vi "Set Colour.vi"(0 "Quick-GUI-Update in":refnum<class "Quick-GUI-Update.lvclass">, 2 "Label":string, 5 "Outer Color":u32(colorbox)=12369084, 9 "Inner Color":u32(colorbox), 11 "Error In":errorcluster) -> (4 "Quick-GUI-Update out":refnum<class "Quick-GUI-Update.lvclass">, 15 "Error Out":errorcluster)   [LabVIEW 2020, in "Easy GUI Operation.lvlib" / "Quick-GUI-Update.lvclass"]
uses:
  Quick-GUI-Update.lvclass
  Quick-GUI-Update.lvclass/Quick-GUI-Update.ctl
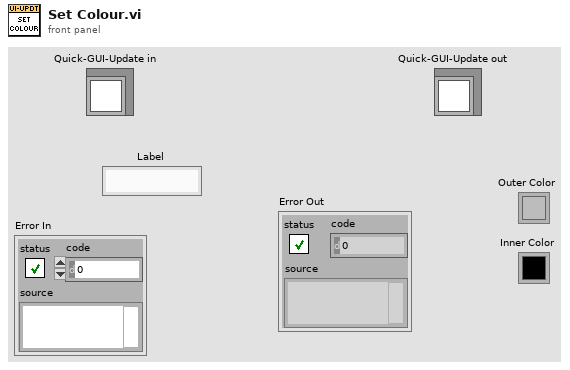
[diagram p1: front panel]
types:
  T1 = map{string, set{cluster{"Ctrl-Ref":refnum<vi>, "Ctrl Index":i32, "Class-Name":string, "Class ID":u32}}}
  T2 = set{cluster{"Ctrl-Ref":refnum<vi>, "Ctrl Index":i32, "Class-Name":string, "Class ID":u32}}
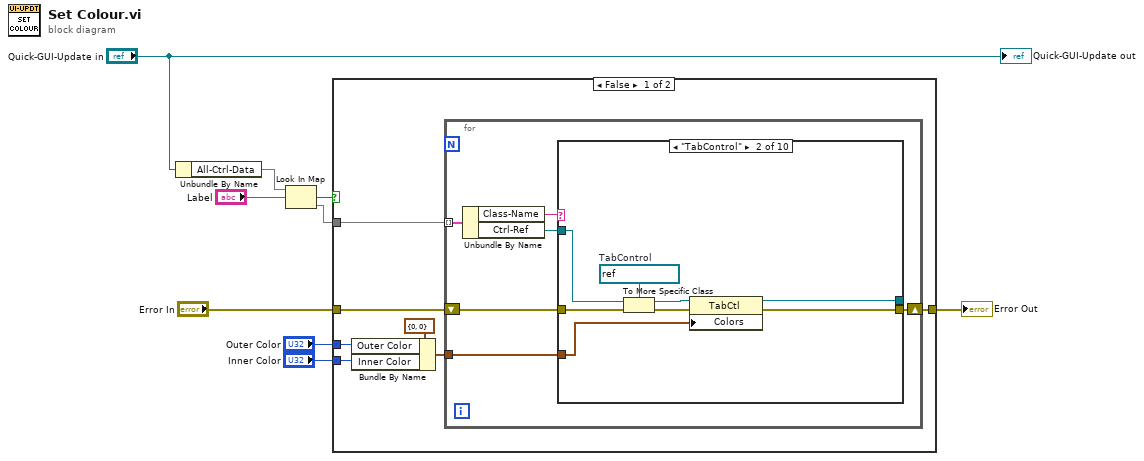
[diagram p0: block diagram]
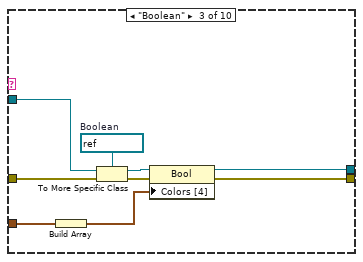
[diagram p3: hidden frame]
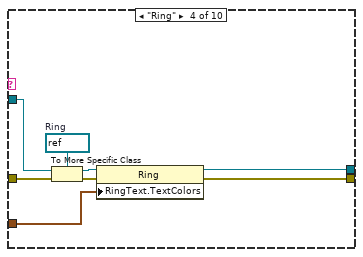
[diagram p4: hidden frame]
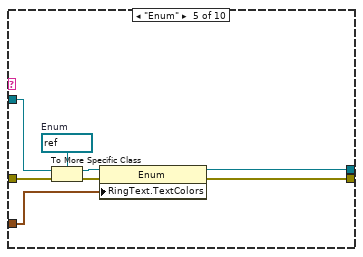
[diagram p5: hidden frame]
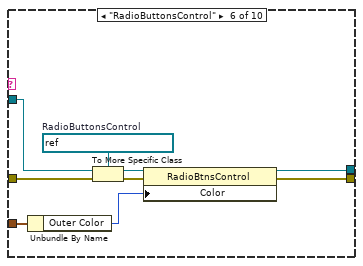
[diagram p6: hidden frame]
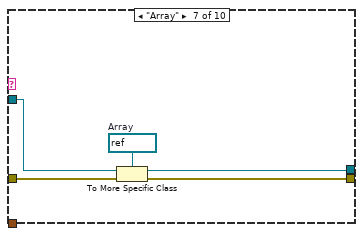
[diagram p7: hidden frame]
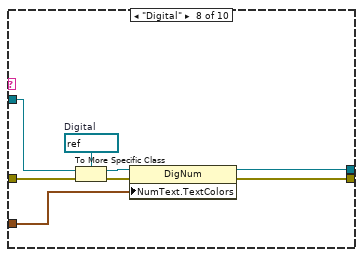
[diagram p8: hidden frame]
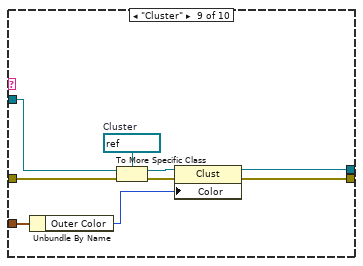
[diagram p9: hidden frame]
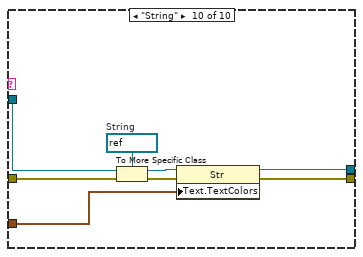
[diagram p10: hidden frame]
diagram:
  n1 = Unbundle By Name("Quick-GUI-Update in") -> ("All-Ctrl-Data"=w4:T1)
  n2 = Look In Map(map=w4, key="Label") -> (key not found?=w1:bool, value=w2:T2)  [unwired: 1 in]
  n3 = case shown="False" w1 {
    tunnel: "Error In" -> [w16 w94]
    tunnel: [w15 w94] -> w8
    tunnel: "Outer Color" -> [w12 _]
    tunnel: "Inner Color" -> [w11 _]
    tunnel: w2 -> [w14 _]
    frame False {
      n4 = Bundle By Name(cluster=cluster{"Outer Color":u32, "Inner Color":u32} {"Outer Color"=0, "Inner Color"=0} ("Color"), "Outer Color"=w12, "Inner Color"=w11) -> (w10:cluster{"Outer Color":u32, "Inner Color":u32})
      n5 = for {
        shift-right: [w21] -> w15
        shift-left: w16 -> [w22]
        tunnel: w14 -> [w20] mode=indexing
        tunnel: w10 -> [w17]
        n6 = Unbundle By Name(w20) -> ("Class-Name"=w19:string, "Ctrl-Ref"=w18:refnum<vi>)
        n7 = case shown="\"TabControl\"" w19 {
          tunnel: w22 -> [w23 w31 w40 w48 w56 w63 w68 w76 w85 w93]
          tunnel: w18 -> [_ w30 w39 w47 w55 w62 w67 w75 w84 w92]
          tunnel: [_ w25 w34 w41 w49 w59 w64 w69 w79 w87] -> _
          tunnel: [w23 w24 w35 w42 w50 w60 w65 w70 w80 w88] -> w21
          tunnel: w17 -> [_ w27 w33 w43 w51 w58 _ w71 w78 w86]
          frame Default {
          }
          frame "TabControl" {
            w29 = refnum<vi> refnum  # TabControl
            n8 = To More Specific Class(target class=w29, reference=w30, error in=w31) -> (specific class reference=w28:refnum<vi>, error out=w26:errorcluster)
            n9 = property class="TabCtl"(reference=w28, error in=w26, "Colors"=w27) -> (reference out=w25:refnum<vi>, error out=w24:errorcluster)
          }
          frame "Boolean" {
            w38 = refnum<vi> refnum  # Boolean
            n10 = Build Array(w33) -> (w32:cluster{"Outer Color":u32, "Inner Color":u32}[])
            n11 = To More Specific Class(target class=w38, reference=w39, error in=w40) -> (specific class reference=w37:refnum<vi>, error out=w36:errorcluster)
            n12 = property class="Bool"(reference=w37, error in=w36, "Colors [4]"=w32) -> (reference out=w34:refnum<vi>, error out=w35:errorcluster)
          }
          frame "Ring" {
            w46 = refnum<vi> refnum  # Ring
            n13 = To More Specific Class(target class=w46, reference=w47, error in=w48) -> (specific class reference=w44:refnum<vi>, error out=w45:errorcluster)
            n14 = property class="Ring"(reference=w44, error in=w45, "RingText.TextColors"=w43) -> (reference out=w41:refnum<vi>, error out=w42:errorcluster)
          }
          frame "Enum" {
            w54 = refnum<vi> refnum  # Enum
            n15 = To More Specific Class(target class=w54, reference=w55, error in=w56) -> (specific class reference=w52:refnum<vi>, error out=w53:errorcluster)
            n16 = property class="Enum"(reference=w52, error in=w53, "RingText.TextColors"=w51) -> (reference out=w49:refnum<vi>, error out=w50:errorcluster)
          }
          frame "RadioButtonsControl" {
            w61 = refnum<vi> refnum  # RadioButtonsControl
            n17 = Unbundle By Name(w58) -> ("Outer Color"=w57:u32)
            n18 = To More Specific Class(target class=w61, reference=w62, error in=w63) -> (specific class reference=w59:refnum<vi>, error out=w60:errorcluster)
            n19 = property class="RadioBtnsControl"(reference=w59, error in=w60, "Color"=w57) -> ()  [unwired: 2 out]
          }
          frame "Array" {
            w66 = refnum<vi> refnum  # Array
            n20 = To More Specific Class(target class=w66, reference=w67, error in=w68) -> (specific class reference=w64:refnum<vi>, error out=w65:errorcluster)
          }
          frame "Digital" {
            w74 = refnum<vi> refnum  # Digital
            n21 = To More Specific Class(target class=w74, reference=w75, error in=w76) -> (specific class reference=w72:refnum<vi>, error out=w73:errorcluster)
            n22 = property class="DigNum"(reference=w72, error in=w73, "NumText.TextColors"=w71) -> (reference out=w69:refnum<vi>, error out=w70:errorcluster)
          }
          frame "Cluster" {
            w83 = refnum<vi> refnum  # Cluster
            n23 = Unbundle By Name(w78) -> ("Outer Color"=w77:u32)
            n24 = To More Specific Class(target class=w83, reference=w84, error in=w85) -> (specific class reference=w82:refnum<vi>, error out=w81:errorcluster)
            n25 = property class="Clust"(reference=w82, error in=w81, "Color"=w77) -> (reference out=w79:refnum<vi>, error out=w80:errorcluster)
          }
          frame "String" {
            w91 = refnum<vi> refnum  # String
            n26 = To More Specific Class(target class=w91, reference=w92, error in=w93) -> (specific class reference=w89:refnum<vi>, error out=w90:errorcluster)
            n27 = property class="Str"(reference=w89, error in=w90, "Text.TextColors"=w86) -> (reference out=w87:refnum<vi>, error out=w88:errorcluster)
          }
        }
      }
    }
    frame True {
    }
  }
  "Error Out" <- w8
  "Quick-GUI-Update out" <- "Quick-GUI-Update in"
